vi "_scope_data.vi"(8 "error in (no error)":errorcluster, 11 "UV-VIS_AVANTES in":refnum<class "UV-VIS_AVANTES.lvclass">) -> (0 "error out":errorcluster, 1 "a_pSpectrum":dbl[](array[numeric]), 2 "a_pTimeLabel":u32, 3 "UV-VIS_AVANTES out":refnum<class "UV-VIS_AVANTES.lvclass">)   [LabVIEW 2018, in "UV-VIS_AVANTES.lvclass"]
uses:
  UV-VIS_AVANTES.lvclass
  C:/Users/Sergey Denisov/Documents/REPS/TRANCON/Classes/Detector/Detector.lvclass
  Detector.lvclass/Detector.ctl
  UV-VIS_AVANTES.lvclass/UV-VIS_AVANTES.ctl
  Detector.lvclass
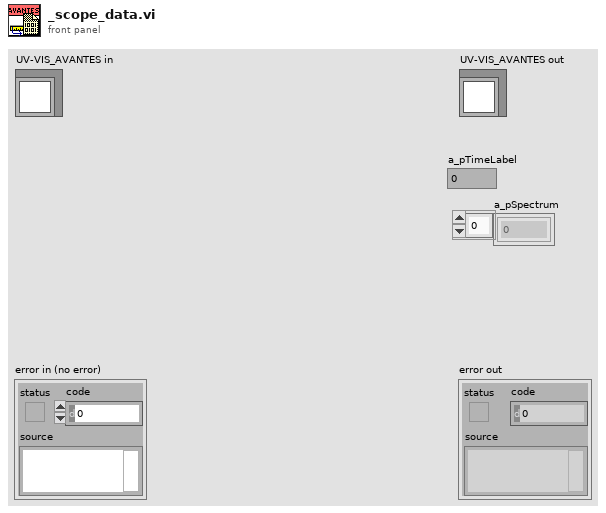
[diagram p1: front panel]
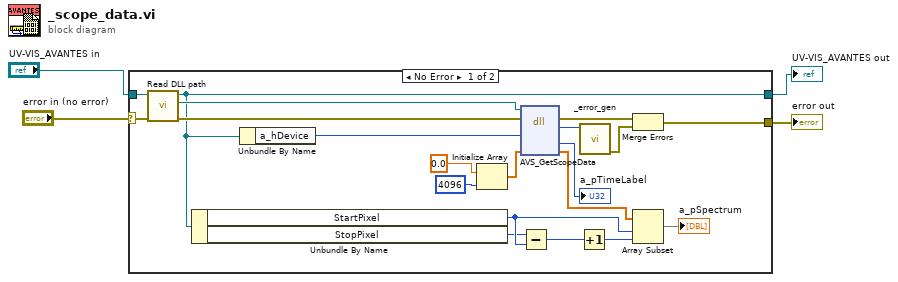
[diagram p0: block diagram]
diagram:
  n1 = case shown="No Error" "error in (no error)" {
    selector: "error in (no error)" -> [w23 w26]
    tunnel: [w22 w26] -> w3
    tunnel: [w11 w25] -> w1
    tunnel: "UV-VIS_AVANTES in" -> [w24 w25]
    frame No Error {
      n2 = call "Read DLL path.vi"("error in (no error)"=w23, "Detector in"=w24) -> ("error out"=w16:errorcluster, "DLL path"=w17:path, "Detector out"=w11:refnum<class "UV-VIS_AVANTES.lvclass">)  [unwired: 7 in]
      n3 = Unbundle By Name(w11) -> ("StartPixel"=w9:u16, "StopPixel"=w8:u16)
      n4 = Unbundle By Name(w11) -> ("a_hDevice"=w15:i32)
      n5 = Initialize Array(0.0 ("element"), 4096 ("dimension size")) -> (w12:dbl[])
      n6 = dll-call lib="C:/AvaSpecX64-DLL_9.4/examples/LabView/LabViewSingleChan/avaspec.dll" fn="AVS_GetScopeData"(path in=w17, error in=w16, "a_hDevice"=w15, "a_pSpectrum"=w12) -> (error out=w18:errorcluster, "return type"=w19:i32, "a_pTimeLabel"=→"a_pTimeLabel":u32, "a_pSpectrum"=w10:dbl[])  [unwired: 3 in, 1 out]
      n7 = Subtract(x=w8, y=w9) -> (x-y=w7:u16)
      n8 = Increment(x=w7) -> (x+1=w6:u16)
      n9 = call "_error_gen.vi"("return type"=w19) -> ("error out"=w21:errorcluster)  [unwired: 10 in]
      n10 = Merge Errors(w18, w21) -> (w22:errorcluster)
      n11 = Array Subset(array=w10, index=w9, length=w6) -> (→"a_pSpectrum":dbl[])
    }
    frame Error {
    }
  }
  "error out" <- w3
  "UV-VIS_AVANTES out" <- w1
